vi "Turner_MasterAquisitionFile_2P.vi"() -> ()   [LabVIEW 2017]
uses:
  <vilib>/userdefined/High Color/IMAQdx.ctl
  <vilib>/vision/driver/IMAQdx.llb/IMAQdx Camera Control Mode.ctl
  <vilib>/vision/driver/IMAQdx.llb/IMAQdx Acquisition Mode.ctl
  <vilib>/vision/driver/IMAQdx.llb/IMAQdx Buffer Number Mode.ctl
  <vilib>/DAQmx/read.llb/DAQmx Read (Digital 1D Bool 1Chan 1Samp).vi
  <vilib>/DAQmx/read.llb/DAQmx Read (Analog 1D Wfm NChan NSamp).vi
  <vilib>/DAQmx/create/channels.llb/DAQmx Create Channel (DI-Digital Input).vi
  <vilib>/DAQmx/miscellaneous.llb/DAQmx Fill In Error Info.vi
  <vilib>/DAQmx/create/channels.llb/DAQmx Create Channel (AI-Voltage-Basic).vi
  <vilib>/DAQmx/configure/timing.llb/DAQmx Timing (Sample Clock).vi
  <vilib>/DAQmx/configure/trigger.llb/DAQmx Start Trigger (Digital Edge).vi
  <vilib>/DAQmx/create/channels.llb/DAQmx Create Channel (CO-Pulse Generation-Frequency).vi
  <vilib>/DAQmx/configure/timing.llb/DAQmx Timing (Implicit).vi
  <vilib>/vision/driver/NI_Vision_Acquisition_Software.lvlib
  <resource>/objmgr/imaqdx.rc
panel:
  out "Data Acquisition - Complete":bool
  out "Acquiring WhiskerCam Data":bool
  out "Acquiring Analog Data":bool
  out "Waiting for MScan Trigger":bool
  in  "MScan Trigger":tag="Dev1/port0/line3"
  out "?":bool[](array[boolean])
  out "Hexadecimal Data":u32 format="%x"
  out "Time Elapsed (Min)":cluster{dbl, dbl}(slide) scale=0.0..5.0
  out "Dropped Frame Table":string[][](table)
  out "Whisker Camera":bool
  out "Analog Data":bool
  out "Analog Acquisition":i32=195617
  in  "Channel Labels":string[](array[string])=["Force_Sensor", "Force_Sensor", "Solenoid_LeftPad", "Solenoid_RightPad", "Solenoid_Auditory", "Respiration", "EMG", "Neural_RH"]
  in  "Physical channels":tag="Dev1/ai2"
  in  "Whisker Cam ID":T1="cam1"
  in  "?":cluster{"Analog Fs":u16}={"Analog Fs"=20000} {"Analog Fs" format="%0.0f"}
  in  "?":cluster{"WhiskerCam Fs":u16}={"WhiskerCam Fs"=150}
  out "Notes Size":i32=6
  out "Notes Reversed":string[](array[string])=["Experimenter", "Animal ID", "Isoflurane time", "Amplifier Gain", "Session ID", "Hemisphere"]
  out "Notes Array":string[](array[string])=["Hemisphere", "Session ID", "Amplifier Gain", "Isoflurane time", "Animal ID", "Experimenter"]
  in  "Notes:":T2={"Experimenter"="Kevin", "Animal ID"="DK11", "Isoflurane time"="1300", "Amplifier Gain"="10000", "Session ID"="Imaging Session One", "Hemisphere"="RH"}
  in  "WhiskerCam Trigger":tag="Dev1/ctr0"
  in  "Target Path":path=path "C:/Users/klt8/Documents/Kevin Test Data/DK11/Habituation Session Two 2.7.19" caption="Final Saved File Location"
  out "Dropped":u32(slide) caption="Dropped WhiskerCam Frames" scale=0.0..50.0
  out "Current File Name":string="190118_14_07_05"
  in  "Time (min)":dbl(knob)=5.0 min=0.5 max=10.0 step=0.5 scale=0.0..5.0 scale format="%#_2g"
  in  "Temp Path":path=path "C:/LabView Test Files" caption="Temporary File Path"
  out "Last Whisk Buffer":u32=1468
  out "Actual WhiskCam Frame Rate":dbl(knob)=150.0 scale=0.0..300.0
  # "Dropped Frames"
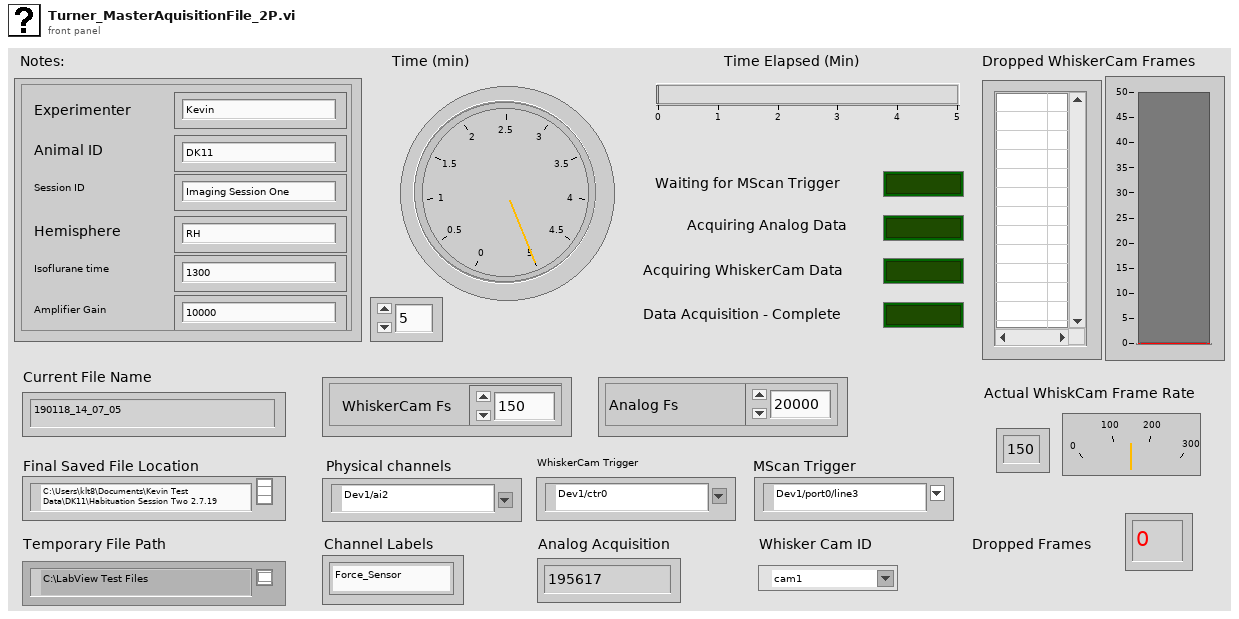
[diagram p1: front panel]
types:
  T1 = typedef "IMAQdx.ctl" = refnum<k21>
  T2 = cluster{"Experimenter":string, "Animal ID":string, "Isoflurane time":string, "Amplifier Gain":string, "Session ID":string, "Hemisphere":string}
  T3 = enum16{"open", "open or create", "create or replace", "create", "open (read-only)"}
  T4 = enum16{"open", "replace", "create", "open or create", "replace or create", "replace or create with confirmation"}
  T5 = typedef "NI_Vision_Acquisition_Software.lvlib/IMAQdx Acquisition Mode.ctl" = enum32{"One Shot", "Continuous"}
  T6 = typedef "NI_Vision_Acquisition_Software.lvlib/IMAQdx Camera Control Mode.ctl" = enum32{"Controller", "Listener"}
  T7 = enum16{"big-endian, network order", "native, host order", "little-endian"}
  T8 = typedef "NI_Vision_Acquisition_Software.lvlib/IMAQdx Buffer Number Mode.ctl" = enum32{"Next", "Last", "Buffer Number", "Every", "Last New"}
  T9 = typedef "Image Type" = u32
  T10 = typedef "IMAQ Image.ctl" = refnum<image>
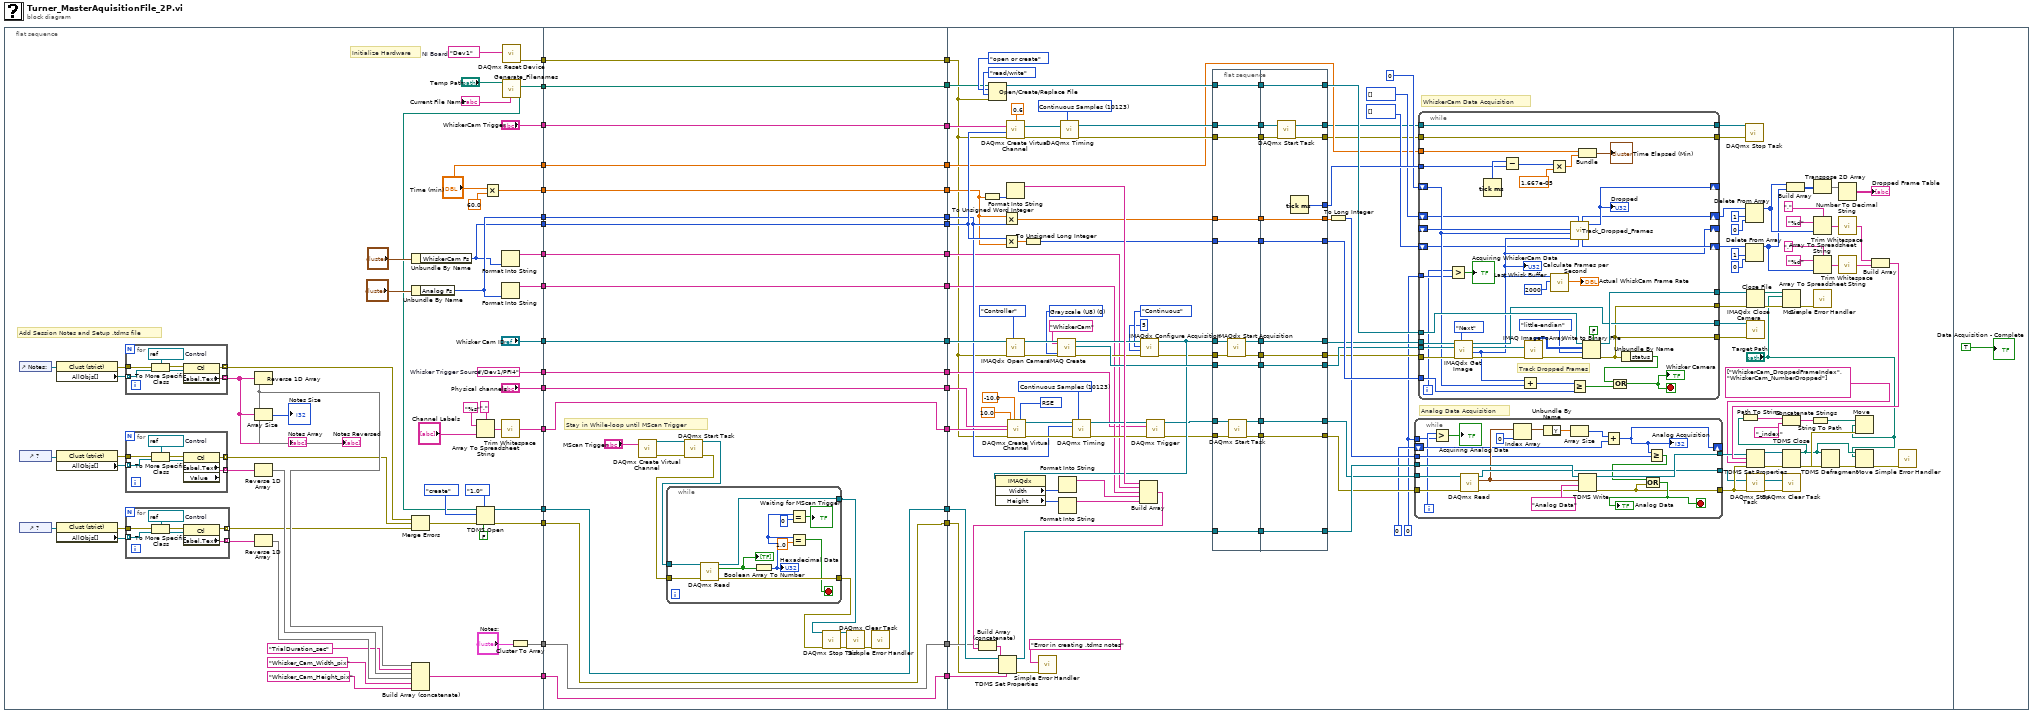
[diagram p0: block diagram]
diagram:
  n1 = flat-sequence {
    tunnel: [w52] -> w17
    tunnel: [w51] -> w16
    tunnel: ["Time (min)"] -> w15
    tunnel: [w49] -> w14
    tunnel: [w48] -> w13
    tunnel: [w47] -> w12
    tunnel: [w46] -> w11
    tunnel: [w45] -> w10
    tunnel: ["WhiskerCam Trigger"] -> w9
    tunnel: [w43] -> w8
    tunnel: ["Physical channels"] -> w7
    tunnel: ["Whisker Cam ID"] -> w6
    tunnel: [w40] -> w5
    tunnel: [w39] -> w4
    tunnel: [w38] -> w3
    tunnel: [w37] -> w2
    tunnel: [w36] -> w1
    tunnel: [w111] -> w34
    tunnel: [w114] -> w33
    tunnel: [w113] -> w32
    tunnel: [w126] -> w31
    tunnel: [w127] -> w30
    tunnel: [w128] -> w29
    tunnel: [w129] -> w28
    tunnel: [w115] -> w27
    tunnel: [w130] -> w26
    tunnel: [w112] -> w25
    tunnel: [w131] -> w24
    tunnel: [w132] -> w23
    tunnel: [w133] -> w22
    tunnel: [w134] -> w21
    tunnel: [w135] -> w20
    tunnel: [w136] -> w19
    tunnel: [w137] -> w18
    tunnel: w17 -> [w137]
    tunnel: w16 -> [w136]
    tunnel: w15 -> [w135]
    tunnel: w14 -> [w134]
    tunnel: w13 -> [w133]
    tunnel: w12 -> [w132]
    tunnel: w11 -> [w131]
    tunnel: w10 -> [w112]
    tunnel: w9 -> [w130]
    tunnel: w8 -> [w115]
    tunnel: w7 -> [w129]
    tunnel: w6 -> [w128]
    tunnel: w5 -> [w127]
    tunnel: w4 -> [w126]
    tunnel: w3 -> [w114]
    tunnel: w2 -> [w113]
    tunnel: w1 -> [w111]
    tunnel: w34 -> [w153]
    tunnel: w33 -> [w158]
    tunnel: w32 -> [w171]
    tunnel: w31 -> [w170]
    tunnel: w30 -> [w156]
    tunnel: w29 -> [w169]
    tunnel: w28 -> [w168]
    tunnel: w27 -> [w167]
    tunnel: w26 -> [w166]
    tunnel: w25 -> [w165]
    tunnel: w24 -> [w164]
    tunnel: w23 -> [w163]
    tunnel: w22 -> [w162]
    tunnel: w21 -> [w161]
    tunnel: w20 -> [w160]
    tunnel: w19 -> [w159]
    tunnel: w18 -> [w157]
    frame #0 {
      w52 = tag "/Dev1/PFI4"  # Whisker Trigger Source
      w59 = tag "Dev1"  # NI Board
      # "Initialize Hardware"
      # "Add Session Notes and Setup .tdms file"
      n2 = control-ref of="Notes:"() -> (w72:refnum<vi>)
      n3 = control-ref of="?"() -> (w70:refnum<vi>)
      n4 = control-ref of="?"() -> (w63:refnum<vi>)
      n5 = property class="Clust (strict)"(reference=w72) -> (error out=w71:errorcluster, "AllObjs[]"=w73:refnum<vi>[])  [unwired: 1 in, 1 out]
      n6 = property class="Clust (strict)"(reference=w70) -> (error out=w68:errorcluster, "AllObjs[]"=w69:refnum<vi>[])  [unwired: 1 in, 1 out]
      n7 = property class="Clust (strict)"(reference=w63) -> (error out=w64:errorcluster, "AllObjs[]"=w66:refnum<vi>[])  [unwired: 1 in, 1 out]
      n8 = for {
        tunnel: [w94] -> w79 mode=indexing
        tunnel: w73 -> [w93] mode=indexing
        tunnel: w71 -> [w92]
        tunnel: [w90] -> w77 mode=indexing
        w95 = refnum<vi> refnum  # Control
        n9 = To More Specific Class(target class=w95, reference=w93, error in=w92) -> (specific class reference=w96:refnum<vi>, error out=w91:errorcluster)
        n10 = property class="Ctl"(reference=w96, error in=w91) -> (error out=w90:errorcluster, "Label.Text"=w94:string)  [unwired: 1 out]
      }
      "Notes Array" <- w79
      n11 = for {
        tunnel: [w101] -> w67 mode=indexing
        tunnel: w69 -> [w100] mode=indexing
        tunnel: w68 -> [w99]
        tunnel: [w97] -> w76 mode=indexing
        w102 = refnum<vi> refnum  # Control
        n12 = To More Specific Class(target class=w102, reference=w100, error in=w99) -> (specific class reference=w103:refnum<vi>, error out=w98:errorcluster)
        n13 = property class="Ctl" props=["Label", "Text", "Value"](reference=w103, error in=w98) -> (error out=w97:errorcluster, "Label.Text"=w101:string)  [unwired: 2 out]
      }
      n14 = for {
        tunnel: [w108] -> w65 mode=indexing
        tunnel: w66 -> [w107] mode=indexing
        tunnel: w64 -> [w106]
        tunnel: [w104] -> w75 mode=indexing
        w109 = refnum<vi> refnum  # Control
        n15 = To More Specific Class(target class=w109, reference=w107, error in=w106) -> (specific class reference=w110:refnum<vi>, error out=w105:errorcluster)
        n16 = property class="Ctl"(reference=w110, error in=w105) -> (error out=w104:errorcluster, "Label.Text"=w108:string)  [unwired: 1 out]
      }
      n17 = Reverse 1D Array(array=w79) -> (reversed array=w80:string[])
      "Notes Reversed" <- w80
      n18 = Array Size(array=w79) -> (size(s)=→"Notes Size":i32)
      n19 = Reverse 1D Array(array=w67) -> (reversed array=w88:string[])
      n20 = Reverse 1D Array(array=w65) -> (reversed array=w89:string[])
      n21 = Unbundle By Name("?") -> ("WhiskerCam Fs"=w46:u16)
      n22 = Unbundle By Name("?") -> ("Analog Fs"=w47:u16)
      n23 = Merge Errors(w77, w76, w75) -> (w78:errorcluster)
      n24 = Build Array (concatenate)(w80, "TrialDuration_sec", w88, w89, "Whisker_Cam_Width_pix", "Whisker_Cam_Height_pix") -> (w36:string[])
      n25 = Array To Spreadsheet String(delimiter (Tab)=",", array="Channel Labels", 3:"%s" ("format string")) -> (spreadsheet string=w83:string)
      n26 = Multiply(x="Time (min)", y=60.0) -> (x*y=w51:dbl)
      n27 = Format Into String(w46) -> (resulting string=w49:string)  [unwired: 3 in, 1 out]
      n28 = Format Into String(w47) -> (resulting string=w48:string)  [unwired: 3 in, 1 out]
      n29 = call <vilib>:"Trim Whitespace.vi"("string"=w83) -> ("trimmed string"=w43:string)  [unwired: 1 in]
      n30 = call <vilib>:"DAQmx Reset Device.vi"("device in"=w59) -> ("error out"=w40:errorcluster)  [unwired: 14 in]
      n31 = call "Generate_Filenames.vi"("path"="Temp Path") -> ("TDMS Path"=w35:path, "Basler Path"=w39:path, "Analog file name"=→"Current File Name":string)  [unwired: 7 in, 1 out]
      n32 = TDMS Open(6:FALSE ("disable buffering? (T)"), 7:enum16{"1.0", "2.0"}."1.0" ("file format version (2.0)"), 8:w78, 10:T3."create" ("operation (0:open)"), 11:w35) -> (0:w38:errorcluster, 3:w37:refnum<k34>)  [unwired: 2 in]
      n33 = Cluster To Array(cluster="Notes:") -> (array=w45:string[])
    }
    frame #1 {
      # "Stay in While-loop until MScan Trigger"
      n34 = call-poly <vilib>:"DAQmx Create Virtual Channel.vi"("lines"="MScan Trigger") -> ("task out"=w120:refnum<k21>, "error out"=w121:errorcluster)  [unwired: 13 in]
      n35 = call <vilib>:"DAQmx Start Task.vi"("task/channels in"=w120, "error in"=w121) -> ("task out"=w125:refnum<k21>, "error out"=w124:errorcluster)  [unwired: 12 in]
      n36 = while {
        tunnel: w125 -> [w147]
        tunnel: w124 -> [w146]
        tunnel: [w144] -> w118
        tunnel: [w145] -> w119
        stop <- w138 stop-if-true
        n37 = call-poly <vilib>:"DAQmx Read.vi"("task/channels in"=w147, "error in"=w146) -> ("task out"=w145:refnum<k21>, "data"=w143:bool[], "error out"=w144:errorcluster)  [unwired: 11 in]
        "?" <- w143
        n38 = Boolean Array To Number(Boolean array=w143) -> (number=w139:u32)
        "Hexadecimal Data" <- w139
        n39 = Equal?(x=w139, y=u32 0) -> (x = y?=→"Waiting for MScan Trigger":bool)
        n40 = Equal?(x=w139, y=1.0) -> (x = y?=w138:bool)
      }
      n41 = call <vilib>:"DAQmx Stop Task.vi"("task/channels in"=w119, "error in"=w118) -> ("task out"=w117:refnum<k21>, "error out"=w116:errorcluster)  [unwired: 12 in]
      n42 = call <vilib>:"DAQmx Clear Task.vi"("task in"=w117, "error in"=w116) -> ("error out"=w123:errorcluster)  [unwired: 13 in]
      n43 = call <vilib>:"Simple Error Handler.vi"("error in (no error)"=w123) -> ()  [unwired: 4 in, 5 out]
    }
    frame #2 {
      w152 = u32 0 ("y")
      w180 = 10123 items=["Finite Samples"=10178, "Continuous Samples"=10123, "Hardware Timed Single Point"=12522] ("sample mode")
      w179 = 10083 items=["default"=-1, "RSE"=10083, "NRSE"=10078, "Differential"=10106, "Pseudodifferential"=12529] ("input terminal configuration")
      w181 = 10123 items=["Finite Samples"=10178, "Continuous Samples"=10123, "Hardware Timed Single Point"=12522] ("sample mode")
      w177 = T9 0 items=["Grayscale (U8)", "Grayscale (I16)", "Grayscale (SGL)", "Complex (CSG)", "RGB (U32)", "HSL (U32)", "RGB (U64)", "Grayscale (U16)"] ("Image Type")
      # "WhiskerCam Data Acquisition"
      # "Analog Data Acquisition"
      n44 = To Unsigned Word Integer(number=w159) -> (unsigned 16bit integer=w242:u16)
      n45 = Open/Create/Replace File(file path (use dialog)=w170, error in=w156, operation (0:open)=T4."open or create", access (0:read/write)=enum16{"read/write", "read-only", "write-only"}."read/write") -> (refnum out=w213:refnum<file>)  [unwired: 2 in, 2 out]
      n46 = Multiply(x=w159, y=w163) -> (x*y=w258:dbl)
      n47 = Multiply(x=w164, y=w159) -> (x*y=w261:dbl)
      n48 = call-poly <vilib>:"DAQmx Create Virtual Channel.vi"("frequency"=w164, "duty cycle"=0.6, "counter"=w166, "error in"=w156) -> ("task out"=w205:refnum<k21>, "error out"=w206:errorcluster)  [unwired: 10 in]
      n49 = Format Into String(w242) -> (resulting string=w271:string)  [unwired: 3 in, 1 out]
      n50 = call <vilib>:"IMAQdx Open Camera.vi"("Camera Control Mode"=IMAQdx_Camera_Control_Mode."Controller", "error in"=w156, "Session In"=w169) -> ("error out"=w203:errorcluster, "Session Out"=w202:T1)  [unwired: 7 in]
      n51 = call-poly <vilib>:"DAQmx Create Virtual Channel.vi"("maximum value"=10.0, "minimum value"=-10.0, "input terminal configuration"=w179, "physical channels"=w168, "name to assign"=w167, "error in"=w156) -> ("task out"=w214:refnum<k21>, "error out"=w215:errorcluster)  [unwired: 8 in]
      n52 = To Unsigned Long Integer(number=w261) -> (unsigned 32bit integer=w262:u32)
      n53 = call "IMAQ Create"("Image Name"="WhiskerCam", "Image Type"=w177, "error in (no error)"=w203) -> ("New Image"=w246:T10, "error out"=w204:errorcluster)  [unwired: 2 in]
      n54 = call-poly <vilib>:"DAQmx Timing.vi"("task/channels in"=w205, "sample mode"=w181, "error in"=w206) -> ("task out"=w224:refnum<k21>, "error out"=w225:errorcluster)  [unwired: 11 in]
      n55 = call-poly <vilib>:"DAQmx Timing.vi"("task/channels in"=w214, "sample mode"=w180, "rate"=w163, "error in"=w215) -> ("task out"=w216:refnum<k21>, "error out"=w217:errorcluster)  [unwired: 10 in]
      n56 = call <vilib>:"IMAQdx Configure Acquisition.vi"("error in"=w204, "Number of Buffers"=u32 5, "Continuous?"=IMAQdx_Acquisition_Mode."Continuous", "Session In"=w202) -> ("error out"=w208:errorcluster, "Session Out"=w245:T1)  [unwired: 6 in]
      n57 = property class="IMAQdx"(reference=w245) -> ("Width"=w243:u32, "Height"=w244:u32)  [unwired: 1 in, 2 out]
      n58 = Format Into String(w243) -> (resulting string=w270:string)  [unwired: 3 in, 1 out]
      n59 = Format Into String(w244) -> (resulting string=w269:string)  [unwired: 3 in, 1 out]
      n60 = Build Array(w271, w161, w162, w270, w269) -> (w272:string[])
      n61 = Build Array (concatenate)(w165, w272) -> (w172:string[])
      n62 = TDMS Set Properties(5:w172, 7:w153, 8:w158, 11:w171) -> (0:w241:errorcluster, 3:w240:refnum<k34>)  [unwired: 2 in, 2 out]
      n63 = call <vilib>:"Simple Error Handler.vi"("error source (\" \")"="Error in creating .tdms notes" ("error source (\" \")"), "error in (no error)"=w241) -> ()  [unwired: 3 in, 5 out]
      n64 = call-poly <vilib>:"DAQmx Trigger.vi"("task/channels in"=w216, "source"=w157, "error in"=w217) -> ("task out"=w218:refnum<k21>, "error out"=w219:errorcluster)  [unwired: 11 in]
      n65 = flat-sequence {
        tunnel: w245 -> [w319]
        tunnel: w208 -> [w318]
        tunnel: [w317] -> w283
        tunnel: [w316] -> w282
        tunnel: [w315] -> w281
        tunnel: w246 -> [w315]
        tunnel: [w314] -> w280
        tunnel: w213 -> [w314]
        tunnel: w218 -> [w313]
        tunnel: w219 -> [w312]
        tunnel: [w311] -> w279
        tunnel: [w310] -> w278
        tunnel: [w309] -> w277
        tunnel: w240 -> [w309]
        tunnel: w224 -> [w308]
        tunnel: [w308] -> w276
        tunnel: w225 -> [w307]
        tunnel: [w307] -> w275
        tunnel: w258 -> [w306]
        tunnel: [w306] -> w274
        tunnel: w262 -> [w305]
        tunnel: [w305] -> w273
        tunnel: [w326] -> w150
        tunnel: [w325] -> w151
        tunnel: [w333] -> w209
        tunnel: w283 -> [w333]
        tunnel: [w332] -> w210
        tunnel: w282 -> [w332]
        tunnel: [w331] -> w211
        tunnel: w281 -> [w331]
        tunnel: [w330] -> w212
        tunnel: w280 -> [w330]
        tunnel: [w329] -> w221
        tunnel: w279 -> [w329]
        tunnel: [w328] -> w220
        tunnel: w278 -> [w328]
        tunnel: [w327] -> w222
        tunnel: w277 -> [w327]
        tunnel: w276 -> [w321]
        tunnel: w275 -> [w324]
        tunnel: w274 -> [w323]
        tunnel: [w323] -> w259
        tunnel: w273 -> [w322]
        tunnel: [w322] -> w268
        tunnel: [w320] -> w201
        frame #0 {
          n66 = call <vilib>:"IMAQdx Start Acquisition.vi"("error in"=w318, "Session In"=w319) -> ("error out"=w316:errorcluster, "Session Out"=w317:T1)  [unwired: 8 in]
          n67 = call <vilib>:"DAQmx Start Task.vi"("task/channels in"=w313, "error in"=w312) -> ("task out"=w311:refnum<k21>, "error out"=w310:errorcluster)  [unwired: 12 in]
        }
        frame #1 {
          n68 = call <vilib>:"DAQmx Start Task.vi"("task/channels in"=w321, "error in"=w324) -> ("task out"=w326:refnum<k21>, "error out"=w325:errorcluster)  [unwired: 12 in]
          n69 = Tick Count (ms)() -> (millisecond timer value=w320:u32)
        }
      }
      n70 = To Long Integer(number=w259) -> (32bit integer=w260:i32)
      n71 = while {
        tunnel: w220 -> [w304]
        tunnel: w221 -> [w303]
        tunnel: w222 -> [w302]
        tunnel: [w301] -> w247
        tunnel: [w288] -> w248
        tunnel: [w300] -> w223
        shift-right: [w293] -> _
        shift-left: 0 -> [w294]
        tunnel: w260 -> [w292]
        tunnel: w152 -> [w284]
        i -> [w285]
        stop <- w289 stop-if-true
        n72 = Greater?(x=w285, y=w284) -> (0:→"Acquiring Analog Data":bool)
        n73 = call-poly <vilib>:"DAQmx Read.vi"("task/channels in"=w303, "error in"=w304) -> ("task out"=w300:refnum<k21>, "data"=w298:waveform(dbl)[], "error out"=w291:errorcluster)  [unwired: 11 in]
        n74 = Index Array(array=w298, index=0) -> (element=w296:waveform(dbl))
        n75 = Unbundle By Name(w296) -> ("Y"=w295:dbl[])
        n76 = Array Size(array=w295) -> (size(s)=w287:i32)
        n77 = TDMS Write(0:w302, 5:"Analog Data" ("group name in (Untitled)"), 9:w298, 11:w291) -> (4:w301:refnum<k34>, 15:w288:errorcluster)  [unwired: 2 in, 2 out]
        n78 = Add(x=w287, y=w294) -> (x+y=w293:i32)
        "Analog Acquisition" <- w293
        n79 = Greater Or Equal?(x=w293, y=w292) -> (x >= y?=w290:bool)
        n80 = Compound Arithmetic op=OR(w288, w290) -> (w289:bool)
        "Analog Data" <- w289
      }
      n81 = while {
        tunnel: [w357] -> w250
        tunnel: [w339] -> w239
        tunnel: [w366] -> w207
        tunnel: w209 -> [w365]
        tunnel: w210 -> [w364]
        tunnel: w211 -> [w363]
        tunnel: w212 -> [w362]
        shift-right: [w356] -> _
        shift-left: _ -> [w361]
        shift-right: [w360] -> _
        shift-left: u32 0 ("New Lost") -> [w355]
        shift-right: [w359] -> w257
        shift-left: u32[] [] ("NewBuffNum") -> [w348]
        shift-right: [w358] -> w226
        shift-left: u32[] [] ("NewNumLost") -> [w349]
        tunnel: w268 -> [w353]
        tunnel: w201 -> [w343]
        tunnel: w160 -> [w341]
        tunnel: [w339] -> w155
        tunnel: w152 -> [w338]
        tunnel: w151 -> [w335]
        tunnel: w150 -> [w334]
        tunnel: [w335] -> w148
        tunnel: [w334] -> w149
        i -> [w337]
        stop <- w350 stop-if-true
        # "Track Dropped Frames"
        n82 = Greater?(x=w337, y=w338) -> (0:→"Acquiring WhiskerCam Data":bool)
        n83 = call <vilib>:"IMAQdx Get Image.vi"("Buffer Number Mode (Next)"=IMAQdx_Buffer_Number_Mode."Next", "error in"=w364, "Image In"=w363, "Session In"=w365) -> ("error out"=w373:errorcluster, "Buffer Number Out"=w356:u32, "Image Out"=w372:T10, "Session Out"=w357:T1)  [unwired: 4 in]
        "Last Whisk Buffer" <- w356
        n84 = Tick Count (ms)() -> (millisecond timer value=w344:u32)
        n85 = Subtract(x=w344, y=w343) -> (x-y=w347:u32)
        n86 = Add(x=w356, y=w355) -> (x+y=w354:u32)
        n87 = call "IMAQ ImageToArray"("error in (no error)"=w373, "Image"=w372) -> ("error out"=w371:errorcluster, "Image Pixels (U8)"=w370:u8[][])  [unwired: 2 in, 3 out]
        n88 = Multiply(x=w347, y=1.667e-05) -> (x*y=w346:dbl)
        n89 = call <vilib>:"Calculate Frames per Second.vi"("Update Interval (ms)"=u32 2000, "Buffer Number"=w356) -> ("Processed Frames/s"=→"Actual WhiskCam Frame Rate":dbl)  [unwired: 7 in, 2 out]
        n90 = call "Track_Dropped_Frames.vi"("NumLost"=w349, "BuffNum"=w348, "Curr Buffer"=w356, "Prev Lost"=w355, "Prev Buffer"=w361) -> ("New Lost"=w360:u32, "NewNumLost"=w358:u32[], "NewBuffNum"=w359:u32[])  [unwired: 4 in]
        "Dropped" <- w360
        n91 = Greater Or Equal?(x=w354, y=w353) -> (x >= y?=w351:bool)
        n92 = Bundle("Time (min)"=w341, w346) -> (→"Time Elapsed (Min)":cluster{"Time (min)":dbl, dbl})  [unwired: 1 in]
        n93 = Write to Binary File(file (use dialog)=w362, data=w370, error in=w371, 5:FALSE ("prepend array or string size? (T)"), 9:T7."little-endian" ("byte order (0:big-endian, network order)")) -> (refnum out=w366:refnum<file>, error out=w339:errorcluster)  [unwired: 1 in, 1 out]
        n94 = Unbundle By Name(w339) -> ("status"=w352:bool)
        n95 = Compound Arithmetic op=OR(w352, w351) -> (w350:bool)
        "Whisker Camera" <- w350
      }
      n96 = call <vilib>:"DAQmx Stop Task.vi"("task/channels in"=w149, "error in"=w148) -> ()  [unwired: 12 in, 2 out]
      n97 = Delete From Array(array=w257, length=1, index=0) -> (array with subset deleted=w267:u32[])  [unwired: 1 out]
      n98 = Delete From Array(array=w226, length=1, index=0) -> (array with subset deleted=w266:u32[])  [unwired: 1 out]
      n99 = Close File(refnum=w207, error in=w239) -> (path=w228:path, error out=w229:errorcluster)
      n100 = call <vilib>:"IMAQdx Close Camera.vi"("error in"=w155, "Session In"=w250) -> ()  [unwired: 9 in, 1 out]
      n101 = call <vilib>:"DAQmx Stop Task.vi"("task/channels in"=w223, "error in"=w248) -> ("task out"=w237:refnum<k21>, "error out"=w238:errorcluster)  [unwired: 12 in]
      n102 = Move(source path=w228, error in=w229, 10:"Target Path") -> (error out=w231:errorcluster)  [unwired: 2 in, 2 out]
      n103 = call <vilib>:"DAQmx Clear Task.vi"("task in"=w237, "error in"=w238) -> ()  [unwired: 13 in, 1 out]
      n104 = Build Array(w267, w266) -> (w263:u32[][])
      n105 = Transpose 2D Array(2D array=w263) -> (transposed array=w264:u32[][])
      n106 = Array To Spreadsheet String(delimiter (Tab)=",", array=w267, 3:"%d" ("format string")) -> (spreadsheet string=w252:string)
      n107 = Array To Spreadsheet String(delimiter (Tab)=",", array=w266, 3:"%d" ("format string")) -> (spreadsheet string=w253:string)
      n108 = call <vilib>:"Simple Error Handler.vi"("error in (no error)"=w231) -> ()  [unwired: 1 in, 8 out]
      n109 = Number To Decimal String(number=w264) -> (decimal integer string=→"Dropped Frame Table":string[][])  [unwired: 1 in]
      n110 = call <vilib>:"Trim Whitespace.vi"("string"=w252) -> ("trimmed string"=w255:string)  [unwired: 1 in]
      n111 = call <vilib>:"Trim Whitespace.vi"("string"=w253) -> ("trimmed string"=w254:string)  [unwired: 1 in]
      n112 = Build Array(w255, w254) -> (w256:string[])
      n113 = TDMS Set Properties(5:w256, 7:string[] ["WhiskerCam_DroppedFrameIndex", "WhiskerCam_NumberDropped"] ("channel name(s) in (Untitled)"), 8:w248, 11:w247) -> (0:w249:errorcluster, 3:w251:refnum<k34>)  [unwired: 2 in, 2 out]
      n114 = TDMS Close(8:w249, 11:w251) -> (0:w227:errorcluster, 3:w233:path)
      n115 = Path To String(path=w233) -> (string=w232:string)
      n116 = Concatenate Strings(w232, "_index" ("string")) -> (w234:string)
      n117 = String To Path(string=w234) -> (path=w235:path)
      n118 = TDMS Defragment(4:w227, 7:w233) -> (0:w236:errorcluster)
      n119 = Move(source path=w235, error in=w236, 10:"Target Path") -> ()  [unwired: 2 in, 3 out]
      n120 = Move(source path=w233, error in=w236, 10:"Target Path") -> (error out=w230:errorcluster)  [unwired: 2 in, 2 out]
      n121 = call <vilib>:"Simple Error Handler.vi"("error in (no error)"=w230) -> ()  [unwired: 1 in, 8 out]
    }
    frame #3 {
      "Data Acquisition - Complete" <- TRUE ("Data Acquisition - Complete")
    }
  }
